vi "Pick Button Hover.vi"(10 "light?":bool, 11 "Background":u32(colorbox)) -> (3 "Color":u32(colorbox))   [LabVIEW 2021, in "Theme.lvclass"]
doc: "perform a calculation to lighten or darken the button to give a hover contrast\n\n<b>Code Developed By:</b> +\nDaniel Coons +\nhttps://github.com/danielcoons/tsc-pop-up"
uses:
  Theme.lvclass
  Theme.lvclass/Theme.ctl
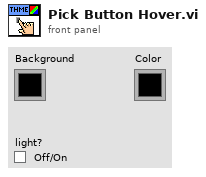
[diagram p1: front panel]
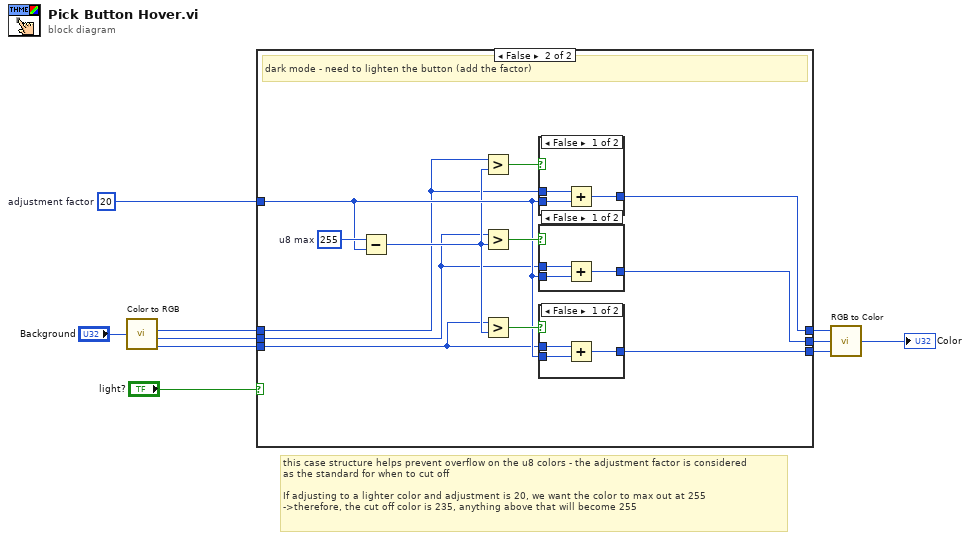
[diagram p0: block diagram]
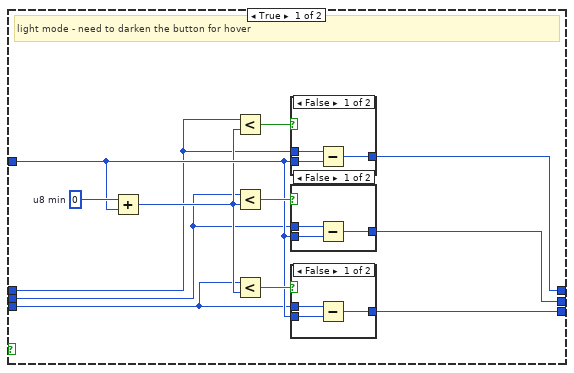
[diagram p2: hidden frame]
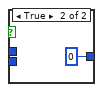
[diagram p3: hidden frame]
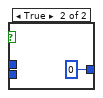
[diagram p4: hidden frame]
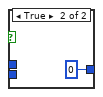
[diagram p5: hidden frame]
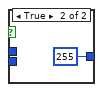
[diagram p6: hidden frame]
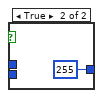
[diagram p7: hidden frame]
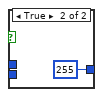
[diagram p8: hidden frame]
diagram:
  w1 = u8 20  # adjustment factor
  # "this case structure helps prevent overflow on the u8 colors - the adjustment factor is considered\nas the standard for when to cut off\n\nIf adjusting to a lighter color and adjustment is 20, we want the color to max out at 255\n->therefore, the cut off color is 235, anything above that will become 255"
  n1 = call <vilib>:"Color to RGB.vi"("Color"="Background") -> ("R"=w3:u8, "G"=w6:u8, "B"=w5:u8)  [unwired: 1 out]
  n2 = case shown="False" "light?" {
    tunnel: [w19 w43] -> w10
    tunnel: [w12 w36] -> w9
    tunnel: [w14 w38] -> w8
    tunnel: w6 -> [w13 w37]
    tunnel: w5 -> [w11 w35]
    tunnel: w3 -> [w15 w39]
    tunnel: w1 -> [w17 w41]
    frame True {
      w18 = u8 0  # u8 min
      # "light mode - need to darken the button for hover"
      n3 = Add(x=w18, y=w17) -> (x+y=w16:u8)
      n4 = Less?(x=w15, y=w16) -> (x < y?=w22:bool)
      n5 = Less?(x=w13, y=w16) -> (x < y?=w21:bool)
      n6 = Less?(x=w11, y=w16) -> (x < y?=w20:bool)
      n7 = case shown="False" w22 {
        tunnel: w17 -> [w33 _]
        tunnel: [w32 u8 0 ("R")] -> w14
        tunnel: w15 -> [w31 _]
        frame False {
          n8 = Subtract(x=w31, y=w33) -> (x-y=w32:u8)
        }
        frame True {
        }
      }
      n9 = case shown="False" w21 {
        tunnel: w17 -> [w29 _]
        tunnel: [w28 u8 0 ("R")] -> w12
        tunnel: w13 -> [w27 _]
        frame False {
          n10 = Subtract(x=w27, y=w29) -> (x-y=w28:u8)
        }
        frame True {
        }
      }
      n11 = case shown="False" w20 {
        tunnel: w17 -> [w25 _]
        tunnel: [w24 u8 0 ("R")] -> w19
        tunnel: w11 -> [w23 _]
        frame False {
          n12 = Subtract(x=w23, y=w25) -> (x-y=w24:u8)
        }
        frame True {
        }
      }
    }
    frame False {
      w42 = u8 255  # u8 max
      # "dark mode - need to lighten the button (add the factor)"
      n13 = Subtract(x=w42, y=w41) -> (x-y=w40:u8)
      n14 = Greater?(x=w39, y=w40) -> (0:w46:bool)
      n15 = Greater?(x=w37, y=w40) -> (0:w45:bool)
      n16 = Greater?(x=w35, y=w40) -> (0:w44:bool)
      n17 = case shown="False" w46 {
        tunnel: w41 -> [w57 _]
        tunnel: [w56 u8 255 ("R")] -> w38
        tunnel: w39 -> [w55 _]
        frame False {
          n18 = Add(x=w55, y=w57) -> (x+y=w56:u8)
        }
        frame True {
        }
      }
      n19 = case shown="False" w45 {
        tunnel: w41 -> [w53 _]
        tunnel: [w52 u8 255 ("R")] -> w36
        tunnel: w37 -> [w51 _]
        frame False {
          n20 = Add(x=w51, y=w53) -> (x+y=w52:u8)
        }
        frame True {
        }
      }
      n21 = case shown="False" w44 {
        tunnel: w41 -> [w49 _]
        tunnel: [w48 u8 255 ("R")] -> w43
        tunnel: w35 -> [w47 _]
        frame False {
          n22 = Add(x=w47, y=w49) -> (x+y=w48:u8)
        }
        frame True {
        }
      }
    }
  }
  n23 = call <vilib>:"RGB to Color.vi"("B"=w10, "G"=w9, "R"=w8) -> ("Color"=→"Color":u32)
